vi "Find ItemID.vi"(8 "error in (no error)":errorcluster, 10 "Item ID":string, 11 "Project Sync Tools in":refnum<class "Project Sync Tools.lvclass">) -> (0 "error out":errorcluster, 1 "Found":bool, 2 "ProjectItem Refnum":refnum<vi>, 3 "CD Build Tools out":refnum<class "Project Sync Tools.lvclass">)   [LabVIEW 2019, in "Project Sync Tools.lvclass"]
uses:
  Project Sync Tools.lvclass
  Project Sync Tools.lvclass/Project Sync Tools.ctl
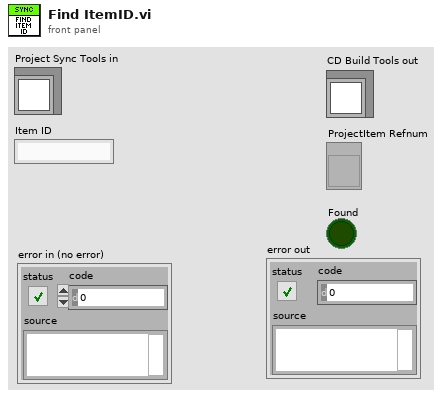
[diagram p1: front panel]
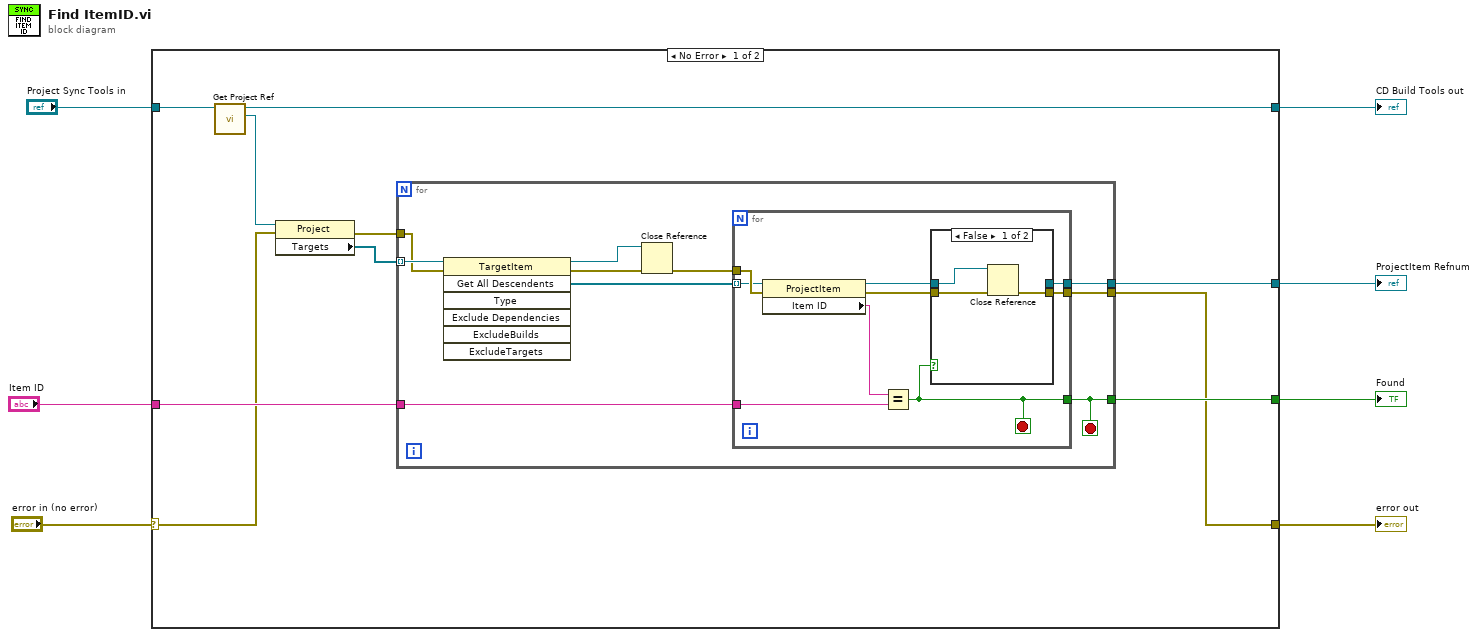
[diagram p0: block diagram]
diagram:
  n1 = case shown="No Error" "error in (no error)" {
    selector: "error in (no error)" -> [w10 w43]
    tunnel: "Item ID" -> [w17 _]
    tunnel: "Project Sync Tools in" -> [w15 w42]
    tunnel: [w14 w42] -> w5
    tunnel: [w13 _] -> w4
    tunnel: [w12 _] -> w3
    tunnel: [w11 w43] -> w2
    frame No Error {
      n2 = call "Get Project Ref.vi"("CD Build Tools in"=w15) -> ("Project Ref"=w8:refnum<vi>, "CD Build Tools out"=w14:refnum<class "Project Sync Tools.lvclass">)  [unwired: 9 in]
      n3 = property class="Project"(reference=w8, error in=w10) -> (error out=w9:errorcluster, "Targets"=w16:refnum<vi>[])  [unwired: 1 out]
      n4 = for {
        tunnel: w16 -> [w22] mode=indexing
        tunnel: w17 -> [w27]
        tunnel: [w26] -> w12
        tunnel: [w25] -> w13
        tunnel: w9 -> [w19]
        tunnel: [w23] -> w11
        stop <- w25 stop-if-true
        n5 = invoke class="TargetItem" method="Get All Descendents"(reference=w22, error in=w19) -> (reference out=w20:refnum<vi>, error out=w18:errorcluster, "All Descendents"=w21:refnum<vi>[])  [unwired: 5 in, 4 out]
        n6 = Close Reference(reference=w20, error in (no error)=w18) -> (error out=w24:errorcluster)
        n7 = for {
          tunnel: w27 -> [w36]
          tunnel: [w30] -> w26
          tunnel: [w33] -> w25
          tunnel: w24 -> [w35]
          tunnel: [w29] -> w23
          tunnel: w21 -> [w28] mode=indexing
          stop <- w33 stop-if-true
          n8 = property class="ProjectItem"(reference=w28, error in=w35) -> (reference out=w31:refnum<vi>, error out=w34:errorcluster, "Item ID"=w32:string)
          n9 = Equal?(x=w32, y=w36) -> (x = y?=w33:bool)
          n10 = case shown="False" w33 {
            tunnel: w34 -> [w39 w41]
            tunnel: w31 -> [w38 w40]
            tunnel: [w37 w41] -> w29
            tunnel: [_ w40] -> w30
            frame False {
              n11 = Close Reference(reference=w38, error in (no error)=w39) -> (error out=w37:errorcluster)
            }
            frame True {
            }
          }
        }
      }
    }
    frame Error {
    }
  }
  "CD Build Tools out" <- w5
  "Found" <- w4
  "ProjectItem Refnum" <- w3
  "error out" <- w2
